vi "Launch Event Loop.vi"(8 "error in (no error)":errorcluster, 11 "ControlArray in":refnum<class "ControlArray.lvclass">) -> (0 "error out":errorcluster, 3 "ControlArray out":refnum<class "ControlArray.lvclass">)   [LabVIEW 2020, in "Control Array.lvlib" / "ControlArray.lvclass"]
uses:
  ControlArray.lvclass
  Event Loop Async.vi
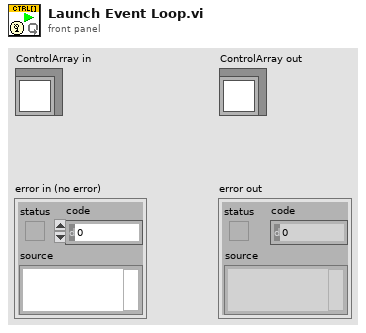
[diagram p1: front panel]
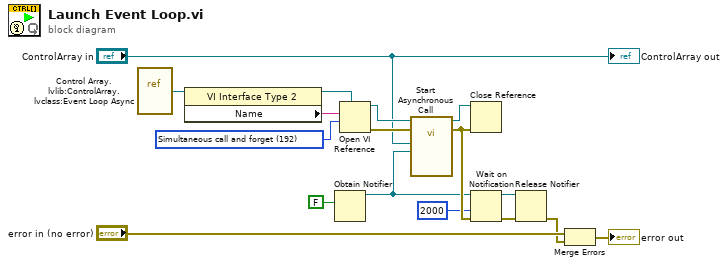
[diagram p0: block diagram]
diagram:
  w10 = 192 items=["Record modifications"=1, "Open templates for editing"=2, "Prompt user to save"=4, "Prepare for reentrant run"=8, "Prompt to find missing subVIs"=16, "Hide loading dialog box"=32, "Enable simultaneous calls"=64, "Prepare to call and forget"=128, "Simultaneous call and forget"=192, "Prepare to call and collect"=256, "Simultaneous call and collect"=320]
  n1 = vi-ref "Control Array.lvlib:ControlArray.lvclass:Event Loop Async.vi"() -> (w8:refnum<vi>)
  n2 = property class="VI Interface Type 2"(reference=w8) -> (reference out=w11:refnum<vi>, "Name"=w9:string)  [unwired: 1 in, 1 out]
  n3 = Obtain Notifier(notification data type=FALSE) -> (notifier out=w6:refnum<notifier>)  [unwired: 3 in, 2 out]
  n4 = Open VI Reference(type specifier VI Refnum (for type only)=w11, vi path=w9, options=w10) -> (vi reference=w13:refnum<vi>, error out=w12:errorcluster)  [unwired: 3 in]
  n5 = call-by-ref "Start Asynchronous Call"(reference=w13, error in=w12, "Handshake"=w6, "ControlArray in"="ControlArray in") -> (reference out=w14:refnum<vi>, error out=w17:errorcluster)  [unwired: 10 in]
  n6 = Close Reference(reference=w14, error in (no error)=w17) -> ()  [unwired: 1 out]
  n7 = Wait on Notification(notifier=w6, timeout in ms (-1)=2000, error in (no error)=w17) -> (notifier out=w4:refnum<notifier>, error out=w3:errorcluster)  [unwired: 1 in, 2 out]
  n8 = Release Notifier(notifier=w4, error in (no error)=w3) -> (error out=w1:errorcluster)  [unwired: 1 in, 2 out]
  n9 = Merge Errors("error in (no error)", w1) -> (→"error out":errorcluster)
  "ControlArray out" <- "ControlArray in"
